vi "Actor Core.vi"(8 "error in":errorcluster, 11 "Beta":refnum<class "Beta.lvclass">) -> (0 "error out":errorcluster, 3 "Actor out":refnum<class "Actor.lvclass">)   [LabVIEW 2018, in "Beta Actor.lvlib" / "Beta.lvclass"]
doc: "This is Actor Core.vi, the main message handling loop for Actors. An actor usually just sits in this loop and processes messages as they arrive. Any error returned by the message Do.vi call will stop the loop, with error code 43 as the canonical signal to stop with no error sent to caller. Descendants may override that in Handle Error.vi."
uses:
  Beta.lvclass
  C:/Program Files (x86)/National Instruments/LabVIEW 2018/vi.lib/ActorFramework/Actor/Actor.lvclass
  <vilib>/ActorFramework/Actor/Actor.lvclass
  <vilib>/ActorFramework/Actor/Actor.lvclass/Actor.ctl
  <vilib>/ActorFramework/Message Enqueuer/Message Enqueuer.lvclass/Message Enqueuer.ctl
  Beta.lvclass/Beta.ctl
  Application Actor/Log Event Msg/Log Event Msg.lvclass/Log Event Msg.ctl
  <vilib>/ActorFramework/Message Enqueuer/Init from Existing Queue.vi
  <vilib>/ActorFramework/Message Enqueuer/Enqueue.vi
  Application Actor/Log Event Msg/Log Event Msg.lvclass
  C:/Program Files (x86)/National Instruments/LabVIEW 2018/vi.lib/ActorFramework/Message/Message.lvclass
  <vilib>/ActorFramework/Message Priority Queue/Priority Enqueue.vi
  <vilib>/ActorFramework/Message Enqueuer/Message Enqueuer.lvclass
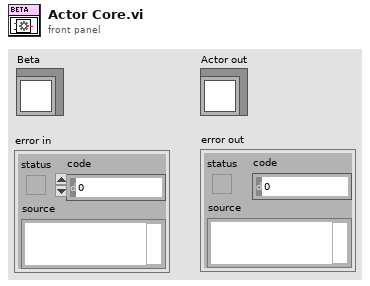
[diagram p1: front panel]
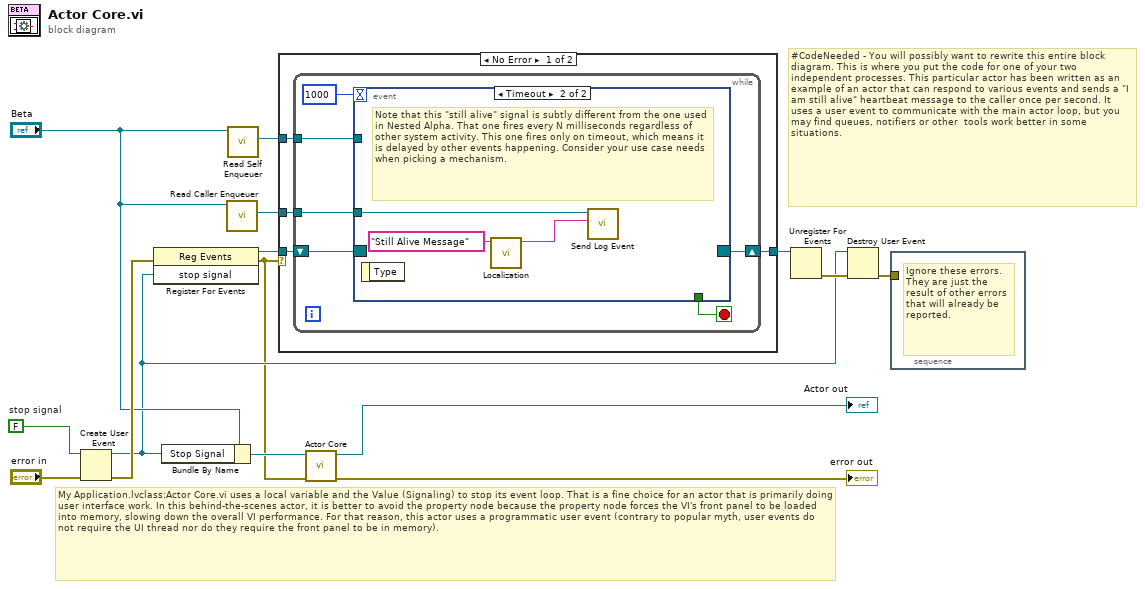
[diagram p0: block diagram]
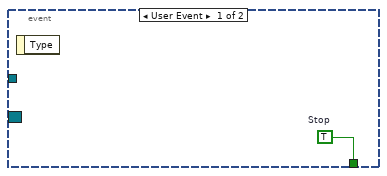
[diagram p2: hidden frame]
diagram:
  w11 = FALSE  # stop signal
  # "My Application.lvclass:Actor Core.vi uses a local variable and the Value (Signaling) to stop its event loop. That is a fine choice for an actor that is primarily doing user interface work. In this behind-the-scenes actor, it is better to avoid the property node because the property node forces the VI's front panel to be loaded into memory, slowing down the overall VI performance. For that reason, this actor uses a programmatic user event (contrary to popular myth, user events do not require the UI thread nor do they require the front panel to be in memory)."
  # "#CodeNeeded - You will possibly want to rewrite this entire block diagram. This is where you put the code for one of your two independent processes. This particular actor has been written as an example of an actor that can respond to various events and sends a \"I am still alive\" heartbeat message to the caller once per second. It uses a user event to communicate with the main actor loop, but you may find queues, notifiers or other  tools work better in some situations."
  n1 = Create User Event(user event datatype=w11, error in="error in") -> (user event=w4:refnum<user-event>, error out=w10:errorcluster)
  n2 = register-events(error in=w10, w4) -> (reference out=w9:refnum<event-registration>, error out=w2:errorcluster)  [unwired: 1 in]
  n3 = Bundle By Name(cluster="Beta", "Stop Signal"=w4) -> (w6:refnum<class "Beta.lvclass">)
  n4 = call <vilib>:"Read Caller Enqueuer.vi"("Actor"="Beta") -> ("Caller Enqueuer"=w13:refnum<class "Message Enqueuer.lvclass">)  [unwired: 10 in]
  n5 = call <vilib>:"Read Self Enqueuer.vi"("Actor"="Beta") -> ("Self Enqueuer"=w14:refnum<class "Message Enqueuer.lvclass">)  [unwired: 10 in]
  n6 = case shown="No Error" w2 {
    tunnel: w14 -> [w19 _]
    tunnel: w13 -> [w18 _]
    tunnel: w9 -> [w17 w30]
    tunnel: [w16 w30] -> w3
    frame No Error {
      n7 = while {
        tunnel: w19 -> [w24]
        tunnel: w18 -> [w23]
        shift-right: [w20] -> w16
        shift-left: w17 -> [w21]
        stop <- w25 stop-if-true
        n8 = event shown="[1] Timeout" {
          selector: w21 -> [_ _]
          dyn-events: [_ _] -> w20
          timeout: 1000 -> [_ _]
          tunnel: [w26 _] -> w25
          tunnel: w24 -> [_ _]
          tunnel: w23 -> [_ w29]
          event User Event {
            w26 = TRUE  # Stop
            n9 = event-data() -> ()  [unwired: 1 in, 1 out]
          }
          event Timeout {
            # "Note that this \"still alive\" signal is subtly different from the one used in Nested Alpha. That one fires every N milliseconds regardless of other system activity. This one fires only on timeout, which means it is delayed by other events happening. Consider your use case needs when picking a mechanism."
            n10 = event-data() -> ()  [unwired: 1 in, 1 out]
            n11 = call "Localization.vi"("Unlocalized"="Still Alive Message") -> ("Localized"=w27:string)  [unwired: 10 in]
            n12 = call "Send Log Event.vi"("Event Text"=w27, "Message Enqueuer"=w29) -> ()  [unwired: 9 in, 1 out]
          }
        }
      }
    }
    frame Error {
    }
  }
  n13 = call-parent "Actor Core.vi"("error in"=w2, "Actor in"=w6) -> ("error out"=→"error out":errorcluster, "Actor out"=→"Actor out":refnum<class "Actor.lvclass">)  [unwired: 8 in]
  n14 = Unregister For Events(event registration refnum=w3) -> (error out=w5:errorcluster)  [unwired: 1 in]
  n15 = Destroy User Event(user event=w4, error in=w5) -> (error out=w1:errorcluster)
  n16 = stacked-sequence {
    tunnel: w1 -> [_]
    frame #0 {
      # "Ignore these errors.\nThey are just the result of other errors that will already be reported."
    }
  }
